vi "ReadCSV.vi"(2 "Reinit":bool, 3 "File Path (.csv)":path) -> (0 "File Open Eror":errorcluster, 1 "Data (index by row)":dbl[][](array[numeric]))   [LabVIEW 2020]
doc: "Reads data from a .csv file. Assumes a header row. Assumes indexing by row. This verison includes error handling if the file is not found."
uses:
  <vilib>/Utility/file.llb/Read Delimited Spreadsheet (DBL).vi
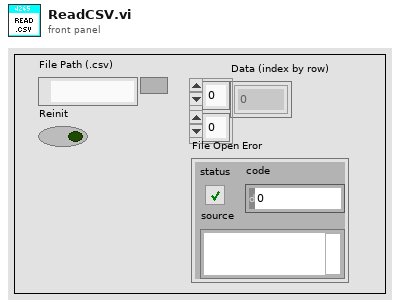
[diagram p1: front panel]
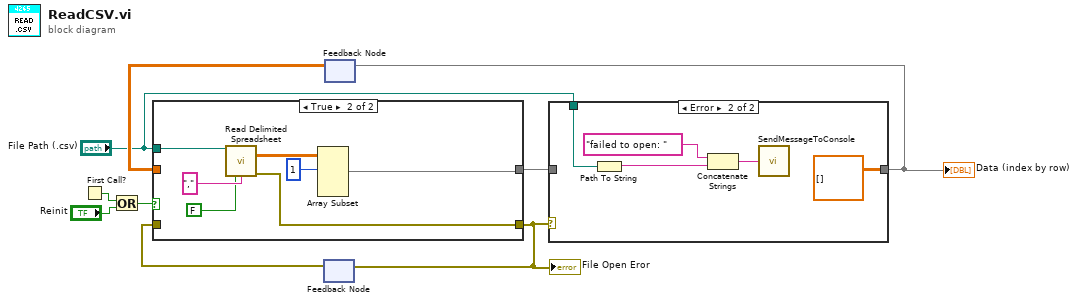
[diagram p0: block diagram]
diagram:
  n1 = First Call?() -> (First Call?: T/F=w7:bool)
  n2 = Or(x=w7, y="Reinit") -> (x .or. y?=w8:bool)
  n3 = feedback #1() -> (w2:errorcluster)  [unwired: 1 in]
  n4 = feedback #2() -> (w9:dbl[][])  [unwired: 1 in]
  n5 = case shown="True" w8 {
    tunnel: "File Path (.csv)" -> [_ w18]
    tunnel: [w11 w14] -> w5
    tunnel: w9 -> [w11 _]
    tunnel: [w10 w12] -> w3
    tunnel: w2 -> [w10 _]
    frame False {
    }
    frame True {
      n6 = call-poly <vilib>:"Read Delimited Spreadsheet.vi"("file path (dialog if empty)"=w18, "transpose? (F)"=FALSE, "delimiter (\\t)"="," ("delimiter (\\t)")) -> ("all rows"=w15:dbl[][], "error out"=w12:errorcluster)  [unwired: 7 in, 4 out]
      n7 = Array Subset(array=w15, index (row)=1 ("index")) -> (w14:dbl[][])  [unwired: 3 in]
    }
  }
  "File Open Eror" <- w3
  n8 = feedback-in #1(w3) -> ()
  n9 = case shown="Error" w3 {
    tunnel: w5 -> [w19 _]
    tunnel: [w19 dbl[][] [] ("Data (index by row)")] -> w4
    tunnel: "File Path (.csv)" -> [_ w23]
    frame No Error {
    }
    frame Error {
      n10 = Path To String(path=w23) -> (string=w22:string)
      n11 = Concatenate Strings("failed to open: " ("string"), w22) -> (w20:string)
      n12 = call "SendMessageToConsole.vi"("Message String"=w20) -> ()  [unwired: 1 in]
    }
  }
  "Data (index by row)" <- w4
  n13 = feedback-in #2(w4) -> ()
